vi "R45_2_realtime.vi"() -> ()   [LabVIEW 2016]
uses:
  <vilib>/rvi/interface/nirviOpenFPGA/nirviOpenFPGA.xnode
  <vilib>/rvi/interface/nirviReadWriteControl/nirviReadWriteControl.xnode
  fpga/R45crio2_fpga.vi
  <vilib>/rvi/errors/niLvFpgaAdjustHostInterfaceError.vi
  <vilib>/rvi/errors/niLvFpgaMergeErrorWithErrorCode.vi
panel:
  out "gfm field":dbl format="%#_8f"
  out "gfm read":u8[](array[numeric])
  out "unsigned byte array 3":u8[](array[numeric])
  out "concatenated string 4":string
  out "Numeric":i32
  out "Timed Out":bool
  out "concatenated string 2":string
  out "unsigned byte array":u8[](array[numeric])
  out "error out 4":errorcluster
  out "Ion gauge 1":u8[](array[numeric])
  out "Convectron 1":u8[](array[numeric])
  out "Ion gauge 2":u8[](array[numeric])
  out "Convectron 2":u8[](array[numeric])
  out "Ion gauge 5":u8[](array[numeric])
  out "Convectron 4":u8[](array[numeric])
  out "Ion gauge 4":u8[](array[numeric])
  out "Convectron 3":u8[](array[numeric])
  in  "Ion gauge cluster control":T1
  in  "Tab Control":enum32{"Contorls", "Read values"}(tab)
  out "X Steerer":dbl(slide) scale=-10.0..10.0 scale format="%#_4g"
  out "ExB 2":dbl(slide) scale=0.0..10.0 scale format="%#_4g"
  out "ExB 1":dbl(slide) scale=0.0..10.0 scale format="%#_4g"
  out "R45 GF magnet faraday cup":bool
  out "R45 GF magnet Aperture":bool
  out "R-45 Aperture 2 IN":bool
  out "R-45 FC2 IN":bool
  out "X steerer readback":fxp<+/-,27,6> format="%.3g"
  out "ExB 1 - voltage monitor":fxp<+/-,26,5> format="%#_3g"
  out "ExB 1 - Current  monitor":fxp<+/-,26,5>
  out "ExB 1+ voltage monitor":fxp<+/-,26,5> format="%#_3g"
  out "ExB +1 Current  monitor":fxp<+/-,26,5>
  out "ExB 2 - voltage monitor":fxp<+/-,26,5>
  out "ExB 2 - Current  monitor":fxp<+/-,26,5>
  out "ExB 2+ voltage monitor":fxp<+/-,26,5>
  out "ExB +2 Current  monitor":fxp<+/-,26,5>
  out "Left voltage monitor":fxp<+/-,26,5> format="%#_3g"
  out "Left Current  monitor":fxp<+/-,26,5> format="%#_3g"
  out "Right voltage monitor":fxp<+/-,26,5> format="%#_3g"
  out "Right Current  monitor":fxp<+/-,26,5> format="%#_3g"
  out "R45 detector Ion gauge cluser 2":T1
  out "R45 waist Ion gauge Cluster 1":T1
  out "exb #1 magnet":dbl
  out "Analog input":fxp<+/-,26,5>[](array[numeric]) format="%#.4g"
  out "gfm set":dbl
  out "gfm read 2":string
  out "cg gauge":bool
  out "ig":bool
  out "exb #1 magnet 2":dbl
  out "ExB 2+":dbl(knob) scale=0.0..10.0 scale format="%#_4g"
  out "ExB 2 -":dbl(knob) scale=0.0..10.0 scale format="%#_4g"
  out "Right":dbl(knob) scale=0.0..10.0 scale format="%#_4g"
  out "Left":dbl(knob) scale=0.0..10.0 scale format="%#_4g"
  out "ExB 1+":dbl(knob) scale=0.0..10.0 scale format="%#_4g"
  out "ExB 1-":dbl(knob) scale=0.0..10.0 scale format="%#_4g"
  out "DIO OUTPUT":bool[](array[boolean])
  # "This controls the # 2 Rio on the right 45   All set and readback \nvalues are unscaled,  so a setting of 5 on a ExB equals 30KV.  \nA setting for 5 on the steerer equals 5kv on the supply\nThe readback module for the dio is not in the rio but can be\n tested next week."
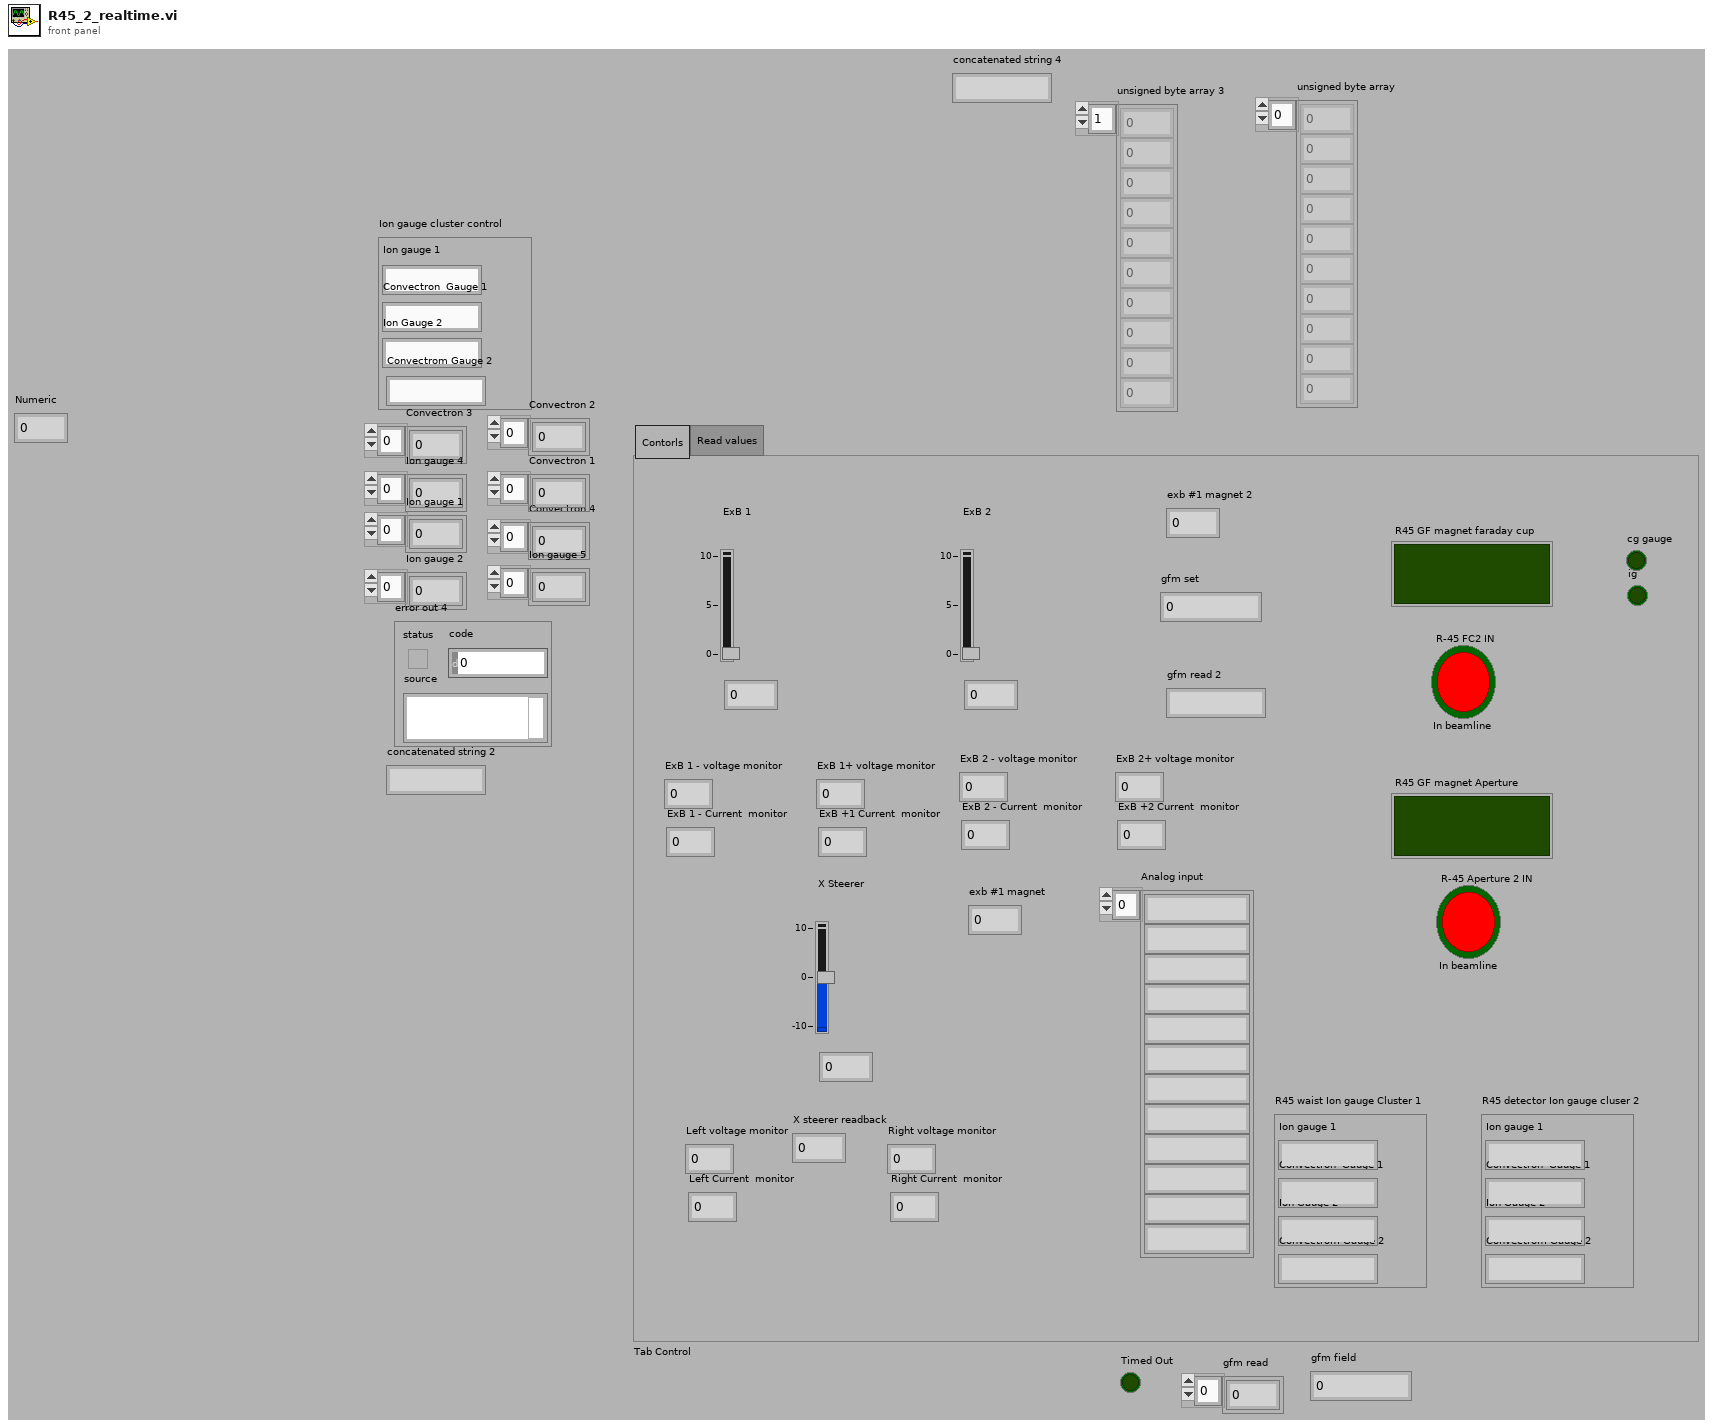
[diagram p1: front panel]
types:
  T1 = cluster{"Ion gauge 1":string, "Convectron  Gauge 1 ":string, "Ion Gauge 2":string, "Convectrom Gauge 2":string}
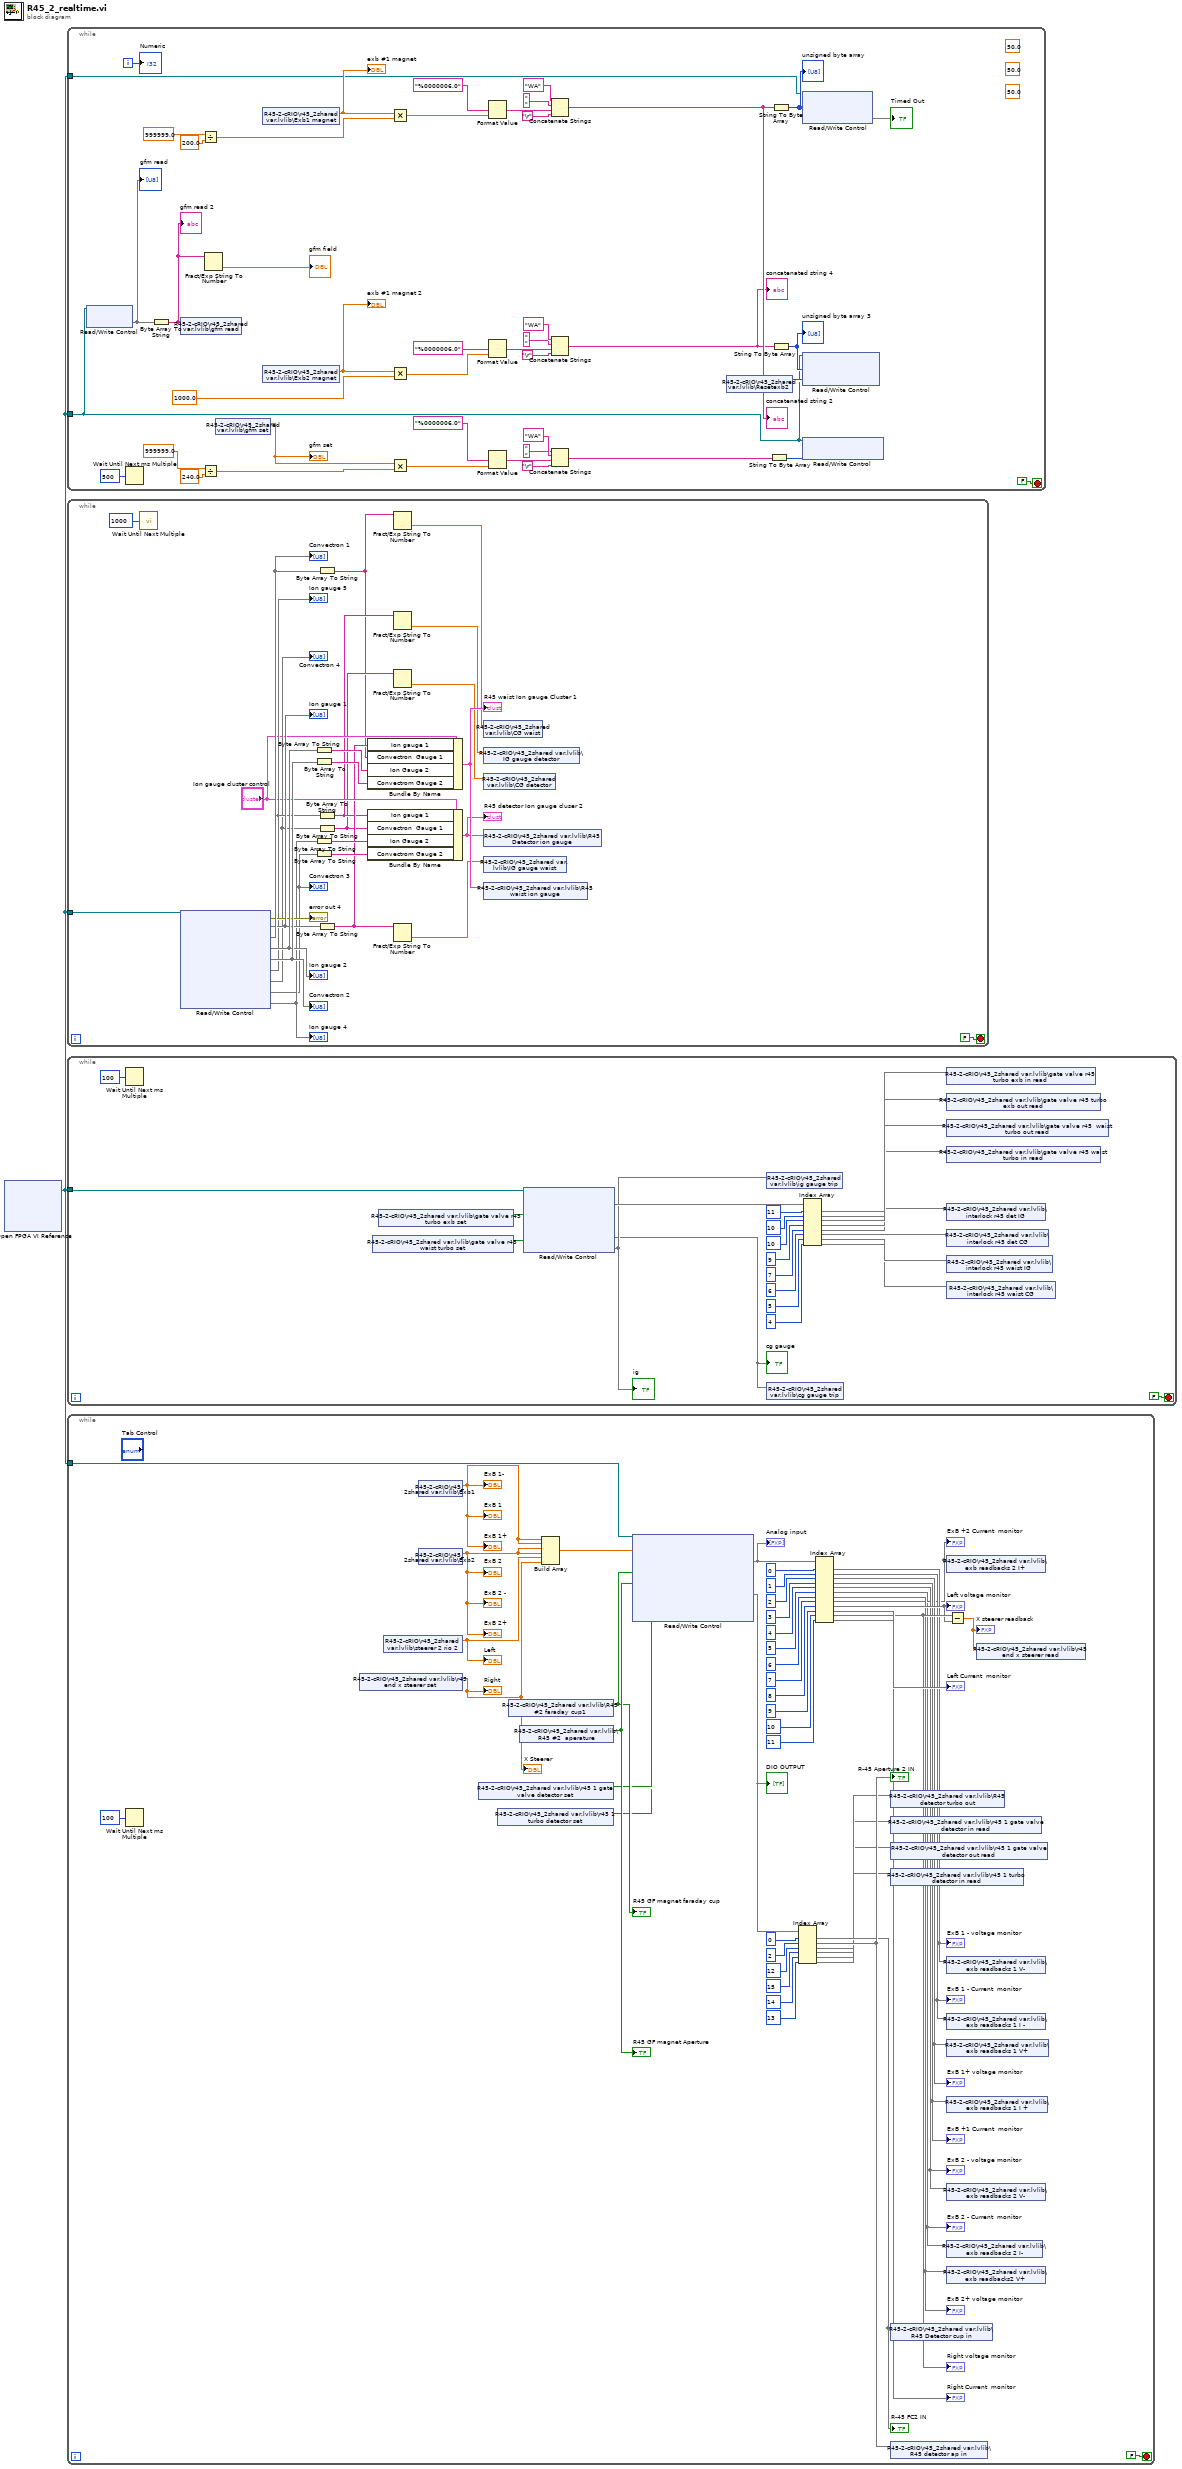
[diagram p0: block diagram]
diagram:
  n1 = xnode "Open FPGA VI Reference"() -> ("FPGA VI Reference Out"=w1:refnum<k20>)  [unwired: 2 in, 1 out]
  n2 = while {
    tunnel: w1 -> [w21]
    tunnel: w1 -> [w8]
    i -> [w20]
    stop <- FALSE stop-if-true
    (unwired) 50.0 ("x")
    (unwired) 50.0 ("x")
    (unwired) 50.0 ("x")
    n3 = xnode "Read/Write Control"("FPGA VI Reference In"=w8) -> ("gfm read"=w7)  [unwired: 1 in, 2 out]
    "gfm read" <- w7
    n4 = Wait Until Next ms Multiple(millisecond multiple=u32 500) -> ()  [unwired: 1 out]
    n5 = Byte Array To String(unsigned byte array=w7) -> (string=w3:string)
    "gfm read 2" <- w3
    n6 = shared-variable "R45-2-cRIO\\r45_2shared var.lvlib\\gfm read"(w3) -> ()  [unwired: 1 in, 1 out]
    n7 = Divide(x=999999.0, y=200.0) -> (x/y=w43:dbl)
    n8 = Divide(x=999999.0, y=240.0) -> (x/y=w12:dbl)
    n9 = Fract/Exp String To Number(string=w3) -> (number=→"gfm field":dbl)  [unwired: 3 in, 1 out]
    n10 = shared-variable "R45-2-cRIO\\r45_2shared var.lvlib\\gfm set"() -> (w4:dbl)  [unwired: 1 in, 1 out]
    "gfm set" <- w4
    n11 = shared-variable "R45-2-cRIO\\r45_2shared var.lvlib\\Exb1 magnet"() -> (w34:dbl)  [unwired: 1 in, 1 out]
    "exb #1 magnet" <- w34
    n12 = shared-variable "R45-2-cRIO\\r45_2shared var.lvlib\\Exb2 magnet"() -> (w24:dbl)  [unwired: 1 in, 1 out]
    "exb #1 magnet 2" <- w24
    n13 = Multiply(x=w34, y=w43) -> (x*y=w41:dbl)
    n14 = Multiply(x=w24, y=1000.0) -> (x*y=w29:dbl)
    n15 = Multiply(x=w4, y=w12) -> (x*y=w14:dbl)
    n16 = Format Value(format string="%0000006.0", value (0)=w41) -> (output string=w38:string)  [unwired: 1 out]
    n17 = Format Value(format string="%0000006.0", value (0)=w29) -> (output string=w26:string)  [unwired: 1 out]
    n18 = Format Value(format string="%0000006.0", value (0)=w14) -> (output string=w17:string)  [unwired: 1 out]
    n19 = Concatenate Strings("WA", " ", w38, "\r") -> (w32:string)
    "concatenated string 2" <- w32
    n20 = Concatenate Strings("WA", " ", w26, "\r") -> (w23:string)
    "concatenated string 4" <- w23
    n21 = Concatenate Strings("WA", " ", w17, "\r") -> (w10:string)
    n22 = shared-variable "R45-2-cRIO\\r45_2shared var.lvlib\\Resetexb2"() -> (w19:bool)  [unwired: 1 in, 1 out]
    n23 = String To Byte Array(string=w10) -> (unsigned byte array=w9:u8[])
    n24 = String To Byte Array(string=w32) -> (unsigned byte array=w35:u8[])
    "unsigned byte array" <- w35
    n25 = String To Byte Array(string=w23) -> (unsigned byte array=w25:u8[])
    "unsigned byte array 3" <- w25
    n26 = xnode "Read/Write Control"("FPGA VI Reference In"=w21, "exb ps set array"=w35) -> ("Timed Out"=→"Timed Out")  [unwired: 1 in, 2 out]
    n27 = xnode "Read/Write Control"("FPGA VI Reference In"=w8, "exb ps set array 2"=w25, "Reset"=w19) -> ()  [unwired: 1 in, 2 out]
    n28 = xnode "Read/Write Control"("FPGA VI Reference In"=w8, "gfm set field array"=w9) -> ()  [unwired: 1 in, 2 out]
    "Numeric" <- w20
  }
  n29 = while {
    tunnel: w1 -> [w56]
    stop <- FALSE stop-if-true
    n30 = call "Wait Until Next Multiple"("Count(mSec)"=u32 1000 ("millisecond multiple")) -> ()  [unwired: 1 out]
    n31 = xnode "Read/Write Control"("FPGA VI Reference In"=w56) -> ("error out"=→"error out 4":errorcluster, "r45 #2 Ion gauge 1"=w67, "r45 #2 Convectron 1"=w68, "r45 #2 Ion gauge 2"=w69, "r45 #2 Convectron 2"=w70, "r45 #3 Ion gauge 1"=w62, "r45 #3 Convectron 1"=w61, "r45 #3 Ion gauge 2"=w59, "r45 #3 Convectron 2"=w60)  [unwired: 1 in, 1 out]
    "Ion gauge 1" <- w67
    "Convectron 1" <- w68
    "Ion gauge 2" <- w69
    "Convectron 2" <- w70
    "Ion gauge 5" <- w62
    "Convectron 4" <- w61
    "Ion gauge 4" <- w60
    "Convectron 3" <- w59
    n32 = Byte Array To String(unsigned byte array=w69) -> (string=w71:string)
    n33 = Byte Array To String(unsigned byte array=w70) -> (string=w72:string)
    n34 = Byte Array To String(unsigned byte array=w60) -> (string=w64:string)
    n35 = Byte Array To String(unsigned byte array=w59) -> (string=w63:string)
    n36 = Byte Array To String(unsigned byte array=w68) -> (string=w49:string)
    n37 = Byte Array To String(unsigned byte array=w62) -> (string=w52:string)
    n38 = Byte Array To String(unsigned byte array=w61) -> (string=w51:string)
    n39 = Byte Array To String(unsigned byte array=w67) -> (string=w53:string)
    n40 = Bundle By Name(cluster="Ion gauge cluster control", "Ion gauge 1"=w53, "Convectron  Gauge 1"=w49, "Ion Gauge 2"=w71, "Convectrom Gauge 2"=w72) -> (w55:T1)
    "R45 waist Ion gauge Cluster 1" <- w55
    n41 = Bundle By Name(cluster="Ion gauge cluster control", "Ion gauge 1"=w52, "Convectron  Gauge 1"=w51, "Ion Gauge 2"=w64, "Convectrom Gauge 2"=w63) -> (w54:T1)
    "R45 detector Ion gauge cluser 2" <- w54
    n42 = Fract/Exp String To Number(string=w49) -> (number=w48:dbl)  [unwired: 3 in, 1 out]
    n43 = Fract/Exp String To Number(string=w52) -> (number=w46:dbl)  [unwired: 3 in, 1 out]
    n44 = Fract/Exp String To Number(string=w51) -> (number=w50:dbl)  [unwired: 3 in, 1 out]
    n45 = Fract/Exp String To Number(string=w53) -> (number=w47:dbl)  [unwired: 3 in, 1 out]
    n46 = shared-variable "R45-2-cRIO\\r45_2shared var.lvlib\\CG waist"(w48) -> ()  [unwired: 1 in, 1 out]
    n47 = shared-variable "R45-2-cRIO\\r45_2shared var.lvlib\\IG gauge detector"(w46) -> ()  [unwired: 1 in, 1 out]
    n48 = shared-variable "R45-2-cRIO\\r45_2shared var.lvlib\\CG detector"(w50) -> ()  [unwired: 1 in, 1 out]
    n49 = shared-variable "R45-2-cRIO\\r45_2shared var.lvlib\\R45 Detector ion gauge"(w54) -> ()  [unwired: 1 in, 1 out]
    n50 = shared-variable "R45-2-cRIO\\r45_2shared var.lvlib\\IG gauge waist"(w47) -> ()  [unwired: 1 in, 1 out]
    n51 = shared-variable "R45-2-cRIO\\r45_2shared var.lvlib\\R45 waist ion gauge"(w55) -> ()  [unwired: 1 in, 1 out]
  }
  n52 = while {
    tunnel: w1 -> [w85]
    stop <- FALSE stop-if-true
    n53 = Wait Until Next ms Multiple(millisecond multiple=u32 100) -> ()  [unwired: 1 out]
    n54 = shared-variable "R45-2-cRIO\\r45_2shared var.lvlib\\gate valve r45  waist turbo set"() -> (w93:bool)  [unwired: 1 in, 1 out]
    n55 = shared-variable "R45-2-cRIO\\r45_2shared var.lvlib\\gate valve r45  turbo exb set"() -> (w92:bool)  [unwired: 1 in, 1 out]
    n56 = xnode "Read/Write Control"("FPGA VI Reference In"=w85, "turbo valve R45 ExB"=w92, "turbo valve r45 waist"=w93) -> ("DIO OUTPUT"=w96, "cg gauge"=w73, "ig"=w74)  [unwired: 1 in, 2 out]
    "cg gauge" <- w73
    "ig" <- w74
    n57 = shared-variable "R45-2-cRIO\\r45_2shared var.lvlib\\ig gauge trip"(w74) -> ()  [unwired: 1 in, 1 out]
    n58 = shared-variable "R45-2-cRIO\\r45_2shared var.lvlib\\cg gauge trip"(w73) -> ()  [unwired: 1 in, 1 out]
    n59 = Index Array(array=w96, index #1=11 ("index"), index #2=10 ("index"), index #3=10 ("index"), index #4=9 ("index"), index #5=7 ("index"), index #6=6 ("index"), index #7=5 ("index"), index #8=4 ("index")) -> (element #1=w75, element #2=w76, element #3=w88, element #4=w87, element #5=w83, element #6=w82, element #7=w78, element #8=w77)
    n60 = shared-variable "R45-2-cRIO\\r45_2shared var.lvlib\\gate valve r45 turbo exb in read"(w75) -> ()  [unwired: 1 in, 1 out]
    n61 = shared-variable "R45-2-cRIO\\r45_2shared var.lvlib\\gate valve r45 turbo exb out read"(w76) -> ()  [unwired: 1 in, 1 out]
    n62 = shared-variable "R45-2-cRIO\\r45_2shared var.lvlib\\gate valve r45  waist turbo out read"(w88) -> ()  [unwired: 1 in, 1 out]
    n63 = shared-variable "R45-2-cRIO\\r45_2shared var.lvlib\\gate valve r45 waist turbo in read"(w87) -> ()  [unwired: 1 in, 1 out]
    n64 = shared-variable "R45-2-cRIO\\r45_2shared var.lvlib\\interlock r45 det IG"(w83) -> ()  [unwired: 1 in, 1 out]
    n65 = shared-variable "R45-2-cRIO\\r45_2shared var.lvlib\\interlock r45 det CG"(w82) -> ()  [unwired: 1 in, 1 out]
    n66 = shared-variable "R45-2-cRIO\\r45_2shared var.lvlib\\interlock r45 waist IG"(w78) -> ()  [unwired: 1 in, 1 out]
    n67 = shared-variable "R45-2-cRIO\\r45_2shared var.lvlib\\interlock r45 waist CG"(w77) -> ()  [unwired: 1 in, 1 out]
  }
  n68 = while {
    tunnel: w1 -> [w146]
    stop <- FALSE stop-if-true
    n69 = Wait Until Next ms Multiple(millisecond multiple=u32 100) -> ()  [unwired: 1 out]
    n70 = shared-variable "R45-2-cRIO\\r45_2shared var.lvlib\\r45 end x steerer set"() -> (w109:dbl)  [unwired: 1 in, 1 out]
    "Right" <- w109
    "X Steerer" <- w109
    n71 = shared-variable "R45-2-cRIO\\r45_2shared var.lvlib\\steerer 2 rio 2"() -> (w108:dbl)  [unwired: 1 in, 1 out]
    "Left" <- w108
    n72 = shared-variable "R45-2-cRIO\\r45_2shared var.lvlib\\Exb1"() -> (w124:dbl)  [unwired: 1 in, 1 out]
    "ExB 1+" <- w124
    "ExB 1-" <- w124
    "ExB 1" <- w124
    n73 = shared-variable "R45-2-cRIO\\r45_2shared var.lvlib\\Exb2"() -> (w112:dbl)  [unwired: 1 in, 1 out]
    "ExB 2 -" <- w112
    "ExB 2+" <- w112
    "ExB 2" <- w112
    n74 = shared-variable "R45-2-cRIO\\r45_2shared var.lvlib\\r45 1 gate valve detector set"() -> (w104:bool)  [unwired: 1 in, 1 out]
    n75 = shared-variable "R45-2-cRIO\\r45_2shared var.lvlib\\r45 1 turbo detector set"() -> (w103:bool)  [unwired: 1 in, 1 out]
    n76 = shared-variable "R45-2-cRIO\\r45_2shared var.lvlib\\R45 #2 faraday cup1"() -> (w113:bool)  [unwired: 1 in, 1 out]
    "R45 GF magnet faraday cup" <- w113
    n77 = shared-variable "R45-2-cRIO\\r45_2shared var.lvlib\\R45 #2  aperature"() -> (w114:bool)  [unwired: 1 in, 1 out]
    "R45 GF magnet Aperture" <- w114
    n78 = Build Array(w124, w124, w112, w112, w108, w109) -> (w145:dbl[])
    n79 = xnode "Read/Write Control"("FPGA VI Reference In"=w146, "Analog Output"=w145, "R45 det  faraday cup"=w113, "R45 det Aperture"=w114, "beamline valve R45 detector"=w104, "turbo valve r45 det turbo"=w103) -> ("Analog input"=w144, "DIO OUTPUT"=w129)  [unwired: 1 in, 2 out]
    "DIO OUTPUT" <- w129
    "Analog input" <- w144
    n80 = Index Array(array=w129, index #1=0 ("index"), index #2=2 ("index"), index #3=12 ("index"), index #4=15 ("index"), index #5=14 ("index"), index #6=13 ("index")) -> (element #1=w110, element #2=w111, element #3=w100, element #4=w98, element #5=w99, element #6=w101)
    "R-45 FC2 IN" <- w110
    "R-45 Aperture 2 IN" <- w111
    n81 = Index Array(array=w144, index #1=0 ("index"), index #2=1 ("index"), index #3=2 ("index"), index #4=3 ("index"), index #5=4 ("index"), index #6=5 ("index"), index #7=6 ("index"), index #8=7 ("index"), index #9=8 ("index"), index #10=9 ("index"), index #11=10 ("index"), index #12=11 ("index")) -> (element #1=w122, element #2=w120, element #3=w123, element #4=w121, element #5=w118, element #6=w116, element #7=w119, element #8=w117, element #9=w125, element #10=→"Left Current  monitor", element #11=w126, element #12=→"Right Current  monitor")
    "ExB 1 - Current  monitor" <- w120
    "ExB 1 - voltage monitor" <- w122
    "ExB +1 Current  monitor" <- w121
    "ExB 1+ voltage monitor" <- w123
    "ExB 2 - voltage monitor" <- w118
    "ExB 2 - Current  monitor" <- w116
    "ExB 2+ voltage monitor" <- w119
    "ExB +2 Current  monitor" <- w117
    "Left voltage monitor" <- w125
    "Right voltage monitor" <- w126
    n82 = shared-variable "R45-2-cRIO\\r45_2shared var.lvlib\\R45 detector turbo out"(w100) -> ()  [unwired: 1 in, 1 out]
    n83 = shared-variable "R45-2-cRIO\\r45_2shared var.lvlib\\r45 1 gate valve detector in read"(w98) -> ()  [unwired: 1 in, 1 out]
    n84 = shared-variable "R45-2-cRIO\\r45_2shared var.lvlib\\r45 1 gate valve detector out read"(w99) -> ()  [unwired: 1 in, 1 out]
    n85 = shared-variable "R45-2-cRIO\\r45_2shared var.lvlib\\r45 1 turbo detector in read"(w101) -> ()  [unwired: 1 in, 1 out]
    n86 = shared-variable "R45-2-cRIO\\r45_2shared var.lvlib\\R45 Detector cup in"(w110) -> ()  [unwired: 1 in, 1 out]
    n87 = shared-variable "R45-2-cRIO\\r45_2shared var.lvlib\\R45 detector ap in"(w111) -> ()  [unwired: 1 in, 1 out]
    n88 = shared-variable "R45-2-cRIO\\r45_2shared var.lvlib\\exb readbacks 2 I+"(w117) -> ()  [unwired: 1 in, 1 out]
    n89 = shared-variable "R45-2-cRIO\\r45_2shared var.lvlib\\exb readbacks 1 V-"(w122) -> ()  [unwired: 1 in, 1 out]
    n90 = shared-variable "R45-2-cRIO\\r45_2shared var.lvlib\\exb readbacks 1 I -"(w120) -> ()  [unwired: 1 in, 1 out]
    n91 = shared-variable "R45-2-cRIO\\r45_2shared var.lvlib\\exb readbacks 1 V+"(w123) -> ()  [unwired: 1 in, 1 out]
    n92 = shared-variable "R45-2-cRIO\\r45_2shared var.lvlib\\exb readbacks 1 I +"(w121) -> ()  [unwired: 1 in, 1 out]
    n93 = shared-variable "R45-2-cRIO\\r45_2shared var.lvlib\\exb readbacks 2 V-"(w118) -> ()  [unwired: 1 in, 1 out]
    n94 = shared-variable "R45-2-cRIO\\r45_2shared var.lvlib\\exb readbacks 2 I-"(w116) -> ()  [unwired: 1 in, 1 out]
    n95 = shared-variable "R45-2-cRIO\\r45_2shared var.lvlib\\exb readbacks2 V+"(w119) -> ()  [unwired: 1 in, 1 out]
    n96 = Subtract(x=w126, y=w125) -> (x-y=w115:dbl)
    "X steerer readback" <- w115
    n97 = shared-variable "R45-2-cRIO\\r45_2shared var.lvlib\\r45 end x steerer read"(w115) -> ()  [unwired: 1 in, 1 out]
  }
